vi "子VI-查看预测结果图.vi"(8 "预测结果路径":path) -> ()   [LabVIEW 2018]
panel:
  out "图片名称":string
  in  "查看图片":bool
  in  "关闭界面":bool
  out "?":T1(plugin-control)
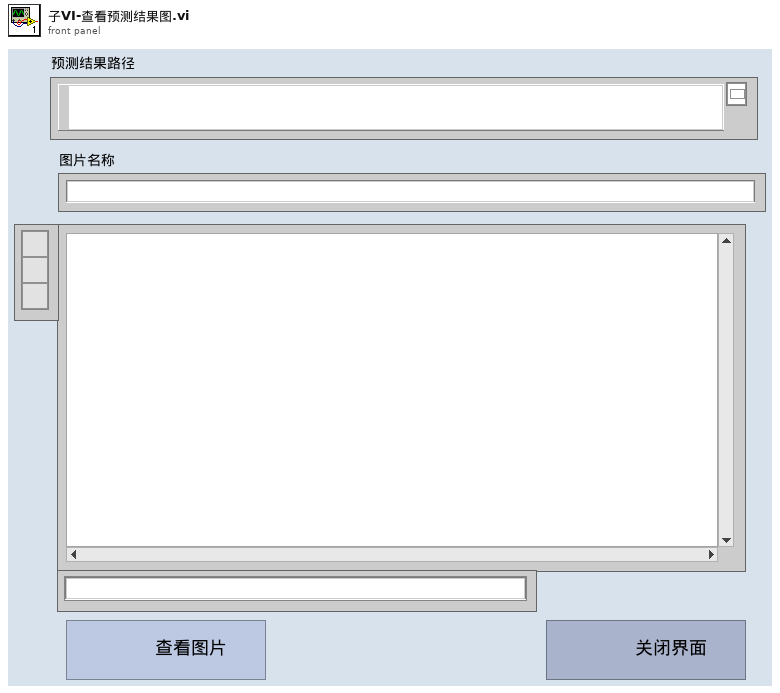
[diagram p1: front panel]
types:
  T1 = typedef "IMAQ Image.ctl" = refnum<image>
  T2 = typedef "Image Type" = u32
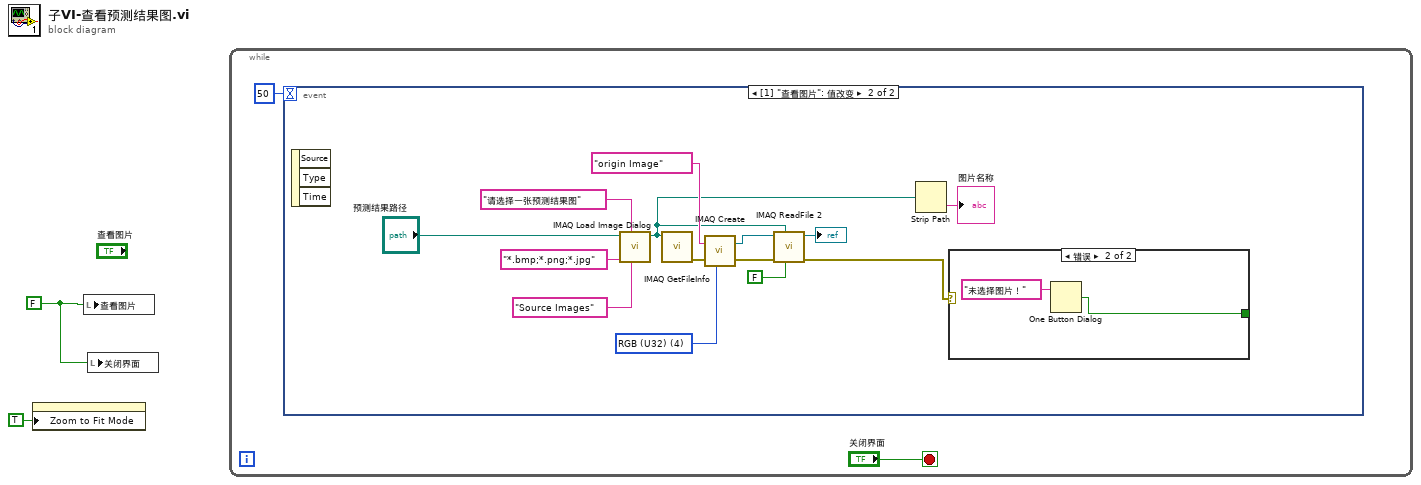
[diagram p0: block diagram]
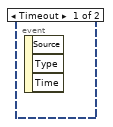
[diagram p2: hidden frame]
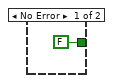
[diagram p3: hidden frame]
diagram:
  w2 = FALSE ("查看图片")
  n1 = property class="ImageControl"("Zoom to Fit Mode"=TRUE) -> ()  [unwired: 2 in, 2 out]
  n2 = local write "查看图片"(w2) -> ()
  n3 = local write "关闭界面"(w2) -> ()
  n4 = while {
    stop <- "关闭界面" stop-if-true
    n5 = event shown="[1] \"查看图片\": 值改变" {
      selector: _ -> [_ _]
      dyn-events: _ -> [_ _]
      timeout: 50 -> [_ _]
      event Timeout {
        n6 = event-data() -> ()  [unwired: 1 in, 3 out]
      }
      event "查看图片": Value Change {
        w8 = T2 4 items=["Grayscale (U8)", "Grayscale (I16)", "Grayscale (SGL)", "Complex (CSG)", "RGB (U32)", "HSL (U32)", "RGB (U64)", "Grayscale (U16)"] ("Image Type")
        n7 = event-data() -> ()  [unwired: 1 in, 3 out]
        n8 = call "IMAQ Load Image Dialog"("Pattern Label"="Source Images", "Prompt"="请选择一张预测结果图" ("prompt"), "Pattern"="*.bmp;*.png;*.jpg", "Start Path"="预测结果路径") -> ("Path"=w6:path)  [unwired: 5 in, 2 out]
        n9 = call "IMAQ GetFileInfo"("File Path"=w6) -> ("error out"=w16:errorcluster)  [unwired: 4 in, 6 out]
        n10 = call "IMAQ Create"("Image Name"="origin Image", "Image Type"=w8, "error in (no error)"=w16) -> ("New Image"=w15:T1, "error out"=w14:errorcluster)  [unwired: 2 in]
        n11 = call "IMAQ ReadFile 2"("Use File Path Image Type"=FALSE, "File Path"=w6, "error in (no error)"=w14, "Image"=w15) -> ("error out"=w7:errorcluster, "Image Out"=→"?":T1)  [unwired: 3 in, 3 out]
        n12 = Strip Path(path=w6) -> (name=→"图片名称":string)  [unwired: 1 out]
        n13 = case shown="错误" w7 {
          tunnel: [FALSE ("true") w20] -> _
          frame No Error {
          }
          frame Error {
            n14 = One Button Dialog(message="未选择图片！" ("消息")) -> (true=w20:bool)  [unwired: 1 in]
          }
        }
      }
    }
  }
